vi "HasRules.vi"(8 "error in (no error)":errorcluster, 11 "CRuleList in":refnum<class "CRuleList.lvclass">) -> (0 "error out":errorcluster, 2 "Has rules?":bool, 3 "CRuleList out":refnum<class "CRuleList.lvclass">)   [LabVIEW 2020, in "DependencyInspection.lvlib" / "CRuleList.lvclass"]
uses:
  CRuleList.lvclass
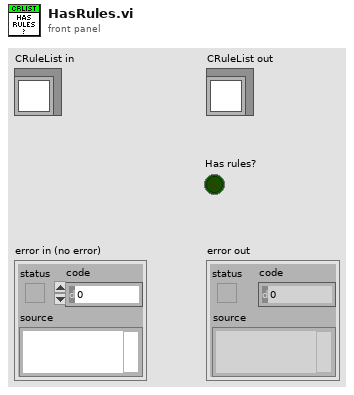
[diagram p1: front panel]
types:
  T1 = typedef "DependencyInspection.lvlib/CRuleList.lvclass/RuleList.ctl" = map{string, refnum<class "IDependencyItemRule.lvclass">}
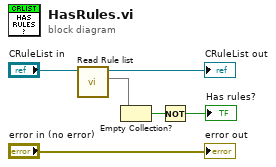
[diagram p0: block diagram]
diagram:
  n1 = call-dynamic "Read Rule list.vi"("CRuleList in"="CRuleList in") -> ("Rule List"=w3:T1, "CRuleList out"=→"CRuleList out":refnum<class "CRuleList.lvclass">)  [unwired: 9 in]
  n2 = Empty Collection?(1:w3) -> (0:w2:bool)
  n3 = Not(x=w2) -> (.not. x?=→"Has rules?":bool)
  "error out" <- "error in (no error)"
